vi "ACT_Loop.vi"() -> ()   [LabVIEW 2023, in "Intake_ACT.lvlib"]
uses:
  Intake_ACT.lvlib
  Cluster_CMD_ACT_Data.ctl
  ENUM_Shooter_Mode.ctl
  Cluster_Shooter Status.ctl
  Type Defs/Cluster_Speed Sensor Values.ctl
  Shooter/Cluster_Velocity Values.ctl
  Shooter/Cluster_Voltage Values.ctl
  ENUM_ACT_State.ctl
  <vilib>/Rock Robotics/WPI/MotorControl/WPI_MotorControlDeviceRef.ctl
  <vilib>/Rock Robotics/WPI/MotorControl/WPI_MotorControlType.ctl
  <vilib>/Rock Robotics/SystemInterfaces/DIO/FPGA_DIOPWMChannel.ctl
  <vilib>/Rock Robotics/WPI/PWM/WPI_PWMDeadband.ctl
  <vilib>/Rock Robotics/SystemInterfaces/DIO/FPGA_DIOChannel.ctl
  <vilib>/Rock Robotics/WPI/ThirdParty/Phoenix-LabVIEW/Motor Controller/Controls/CTRE_Phoenix_MotorControl_ControlMode.ctl
  ENUM_ACT_Action.ctl
  <vilib>/Rock Robotics/WPI/ThirdParty/Phoenix-LabVIEW/Motor Controller/Controls/CTRE_Phoenix_MotorControl_TalonFXInvertType.ctl
  <vilib>/Rock Robotics/WPI/ThirdParty/Phoenix-LabVIEW/Motor Controller/Controls/CTRE_Phoenix_MotorControl_NeutralMode.ctl
  RoboRIO Utilities/Global_STOP.vi
  Global_CMD_ACT_Data In.vi
  Global_ACT_Data Out.vi
  Shooter/Shooter_ACT.lvlib
panel:
  out "Motor Status":T1
  out "Target RPM":dbl
  out "Input DBL Data":T5
  out "Output DBL Data":dbl
  out "Cycle Time (S)":dbl format="%.3g"
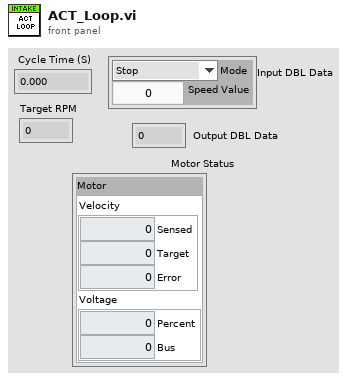
[diagram p1: front panel]
types:
  T1 = typedef "Intake_ACT.lvlib/Cluster_Shooter Status.ctl" = cluster{"Motor":T2}
  T2 = typedef "Cluster_Speed Sensor Values.ctl" = cluster{"Velocity":T3, "Voltage":T4}
  T3 = typedef "Shooter_ACT.lvlib/Cluster_Velocity Values.ctl" = cluster{"Sensed":dbl, "Target":dbl, "Error":dbl}
  T4 = typedef "Shooter_ACT.lvlib/Cluster_Voltage Values.ctl" = cluster{"Percent":dbl, "Bus":dbl}
  T5 = typedef "Intake_ACT.lvlib/Cluster_CMD_ACT_Data.ctl" = cluster{"Mode":T6, "Speed Value":dbl}
  T6 = typedef "Intake_ACT.lvlib/ENUM_Shooter_Mode.ctl" = enum16{"Stop", "Speed Percent", "Speed RPM"}
  T7 = typedef "CTRE_Phoenix_MotorControl_ControlMode.ctl" = u16
  T8 = typedef "WPI_MotorControlDeviceRef.ctl" = cluster{"DeviceStatus":errorcluster, "Type":T9, "PWM":cluster{"PWM Channel":T10, "DeadBand":T11}, "CAN":cluster{"Device Number":u8, "SetOutput VI Ref":variant, "GetOutput VI Ref":variant, "Enable VI Ref":variant, "Disable VI Ref":variant, "Data":variant}, "Invert":bool, "DIO PWM":cluster{"PWM \"Enable\" Channel":T10, "DIOChannel":T12, "PWM Rate":dbl}}
  T9 = typedef "WPI_MotorControlType.ctl" = enum16{"PWM", "CAN", "DIO PWM"}
  T10 = typedef "FPGA_DIOPWMChannel.ctl" = enum8{"PWM 0", "PWM 1", "PWM 2", "PWM 3", "PWM 4", "PWM 5", "PWM 6", "PWM 7", "PWM 8", "PWM 9", "PWM MXP 0", "PWM MXP 1", "PWM MXP 2", "PWM MXP 3", "PWM MXP 4", "PWM MXP 5", "PWM MXP 6", "PWM MXP 7", "PWM MXP 8", "PWM MXP 9", "Invalid"}
  T11 = typedef "WPI_PWMDeadband.ctl" = cluster{"Name":string, "maxPositivePwm":i32, "minPositivePwm":i32, "centerPwm":i32, "maxNegativePwm":i32, "minNegativePwm":i32, "angularRange":u16}
  T12 = typedef "FPGA_DIOChannel.ctl" = enum8{"DIO 0", "DIO 1", "DIO 2", "DIO 3", "DIO 4", "DIO 5", "DIO 6", "DIO 7", "DIO 8", "DIO 9", "DIO MXP 0", "DIO MXP 1", "DIO MXP 2", "DIO MXP 3", "DIO MXP 4", "DIO MXP 5", "DIO MXP 6", "DIO MXP 7", "DIO MXP 8", "DIO MXP 9", "DIO MXP 10", "DIO MXP 11", "DIO MXP 12", "DIO MXP 13", "DIO MXP 14", "DIO MXP 15", "SPI Port CS1", "SPI Port CS2", "SPI Port CS3", "SPI Port MISO", "SPI Port MOSI", "Invalid"}
  T13 = typedef "Intake_ACT.lvlib/ENUM_ACT_State.ctl" = enum16{"Starting", "Stopping", "Intaking", "Shutdown"}
  T14 = typedef "Intake_ACT.lvlib/ENUM_ACT_Action.ctl" = enum16{"No Action", "Reset Time", "Reset All", "Setup Motors", "Setup Sensors", "Stop", "Set Speed RPM", "Set Speed Percent"}
  T15 = cluster{"Motor Ref":T8, "State":T13, "Previous State":T13, "Current Time":timestamp, "Previous Time":timestamp, "Start Time":timestamp, "Target Time (ms)":u32, "Cycle Time(S)":dbl, "ACT Input":T5, "Motor Value":dbl, "Control Mode":T7, "Target RPM":dbl, "Motor Status":T1, "ACT Input from Shooter":T5}
  T16 = typedef "CTRE_Phoenix_MotorControl_NeutralMode.ctl" = enum8{"EEPROMSetting", "Override to Coast", "Override to Brake"}
  T17 = typedef "CTRE_Phoenix_MotorControl_TalonFXInvertType.ctl" = enum16{"Counter-Clockwise", "Clockwise"}
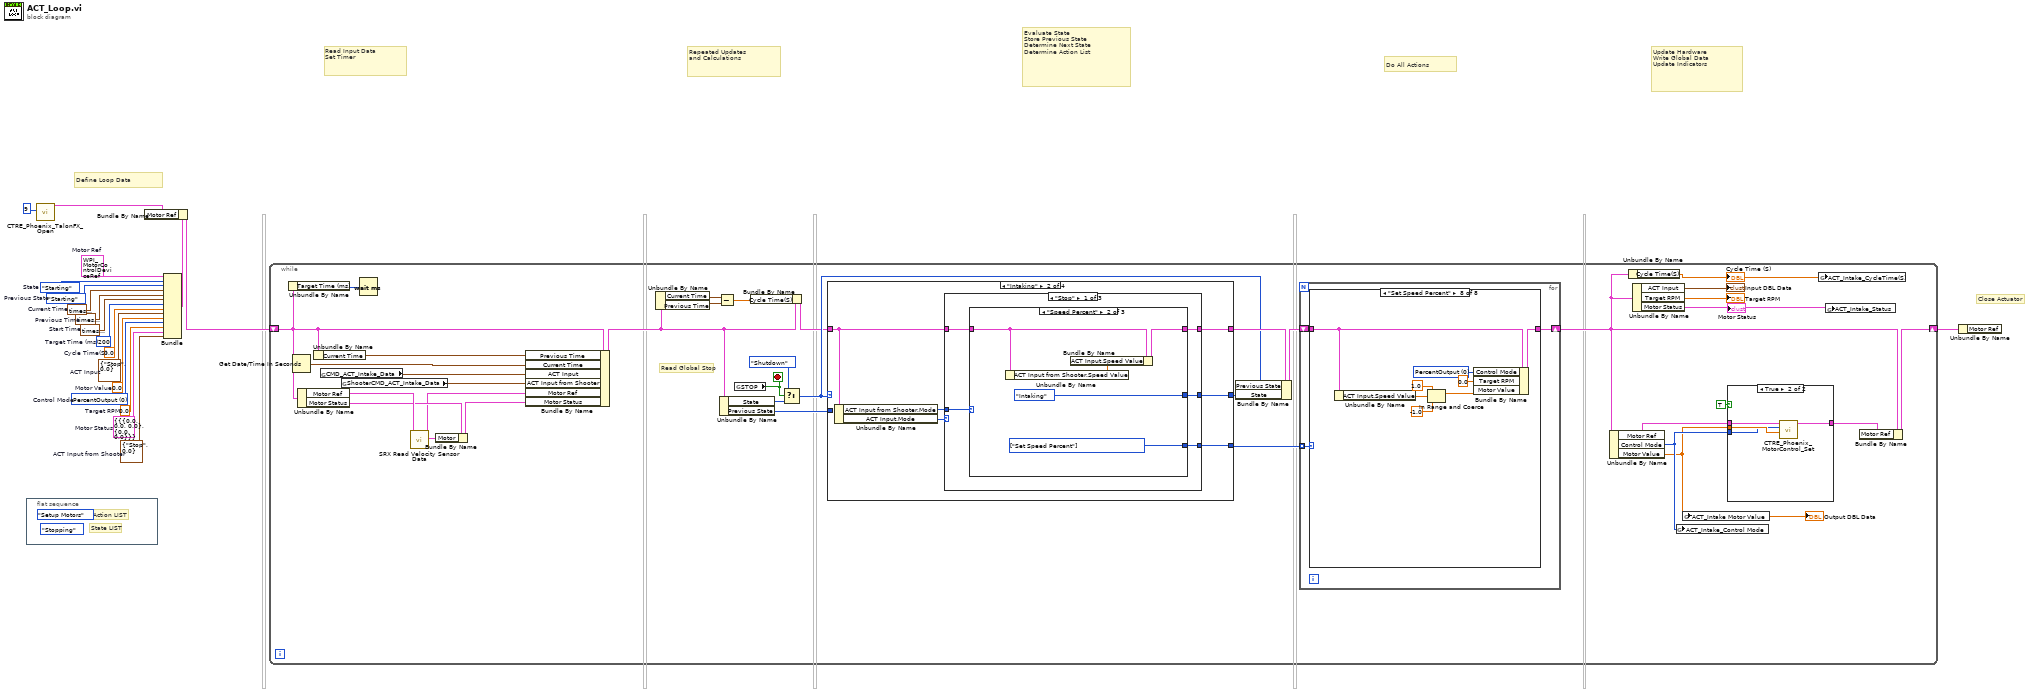
[diagram p0: block diagram]
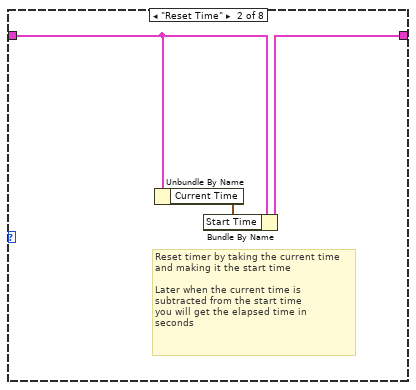
[diagram p4: hidden frame]
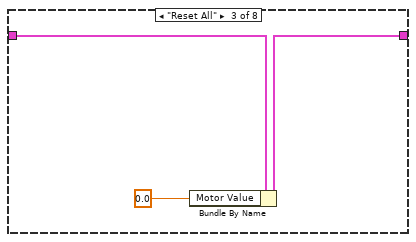
[diagram p5: hidden frame]
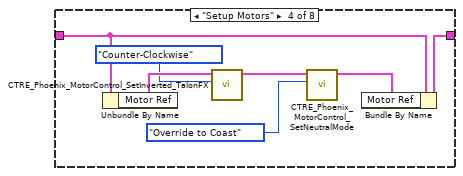
[diagram p6: hidden frame]
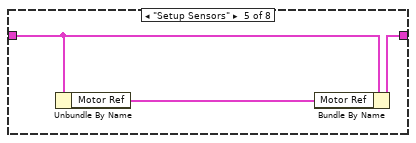
[diagram p7: hidden frame]
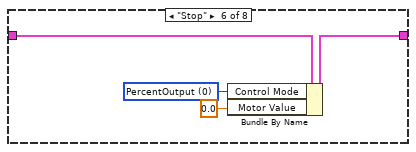
[diagram p8: hidden frame]
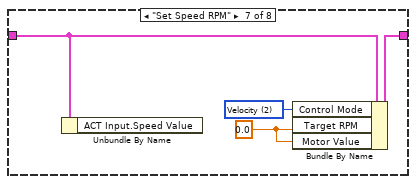
[diagram p9: hidden frame]
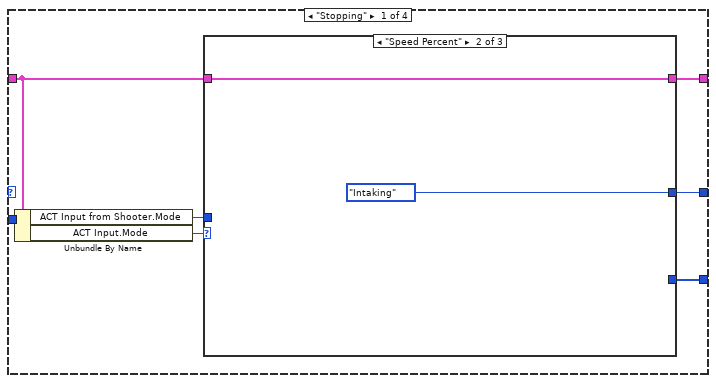
[diagram p10: hidden frame]
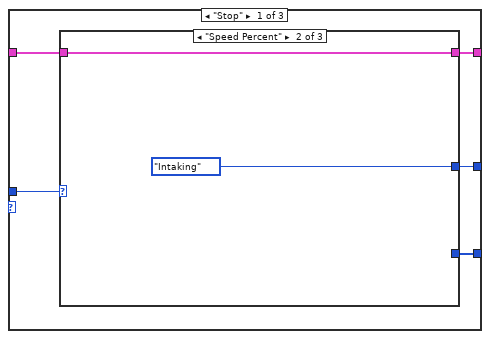
[diagram p11: hidden frame]
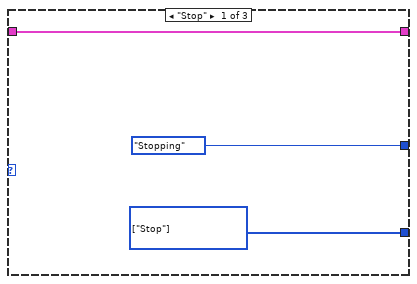
[diagram p12: hidden frame]
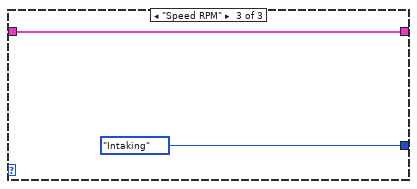
[diagram p13: hidden frame]
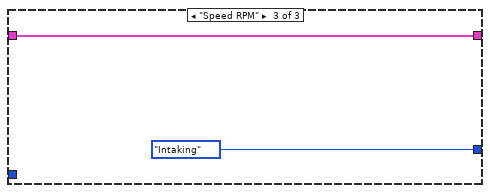
[diagram p14: hidden frame]
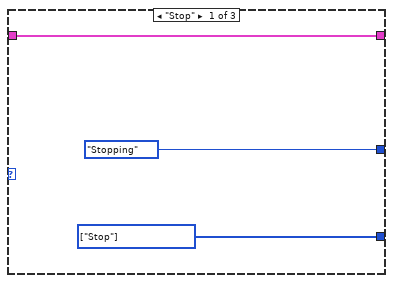
[diagram p15: hidden frame]
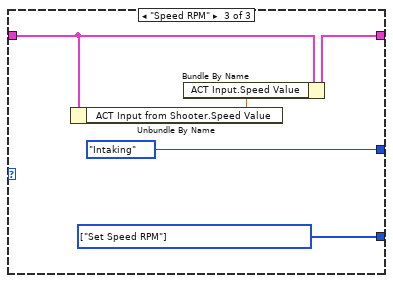
[diagram p16: hidden frame]
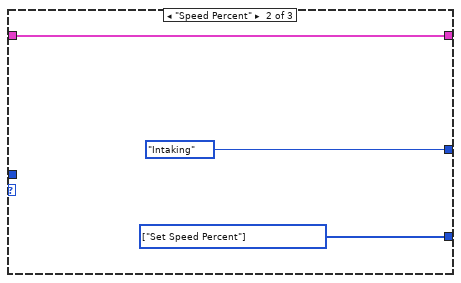
[diagram p17: hidden frame]
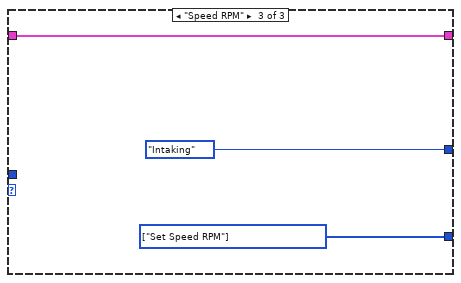
[diagram p18: hidden frame]
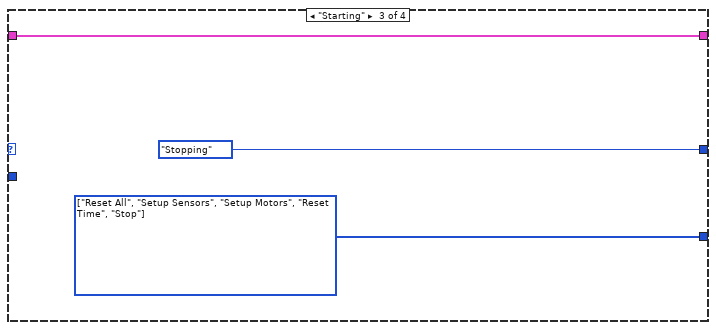
[diagram p19: hidden frame]
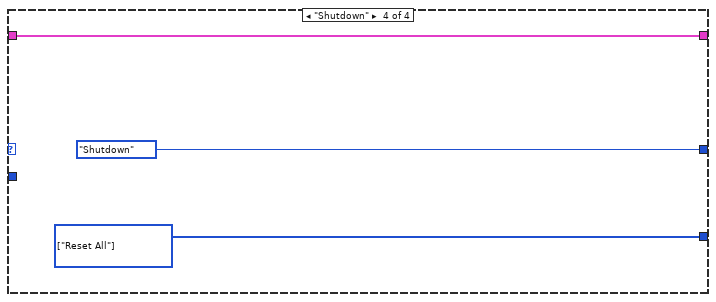
[diagram p20: hidden frame]
diagram:
  w1 = T5 {"Mode"=enum."Stop", "Speed Value"=0.0}  # ACT Input from Shooter
  w2 = T7 0 items=["PercentOutput"=0, "Position"=1, "Velocity"=2, "Current"=3, "Follower"=5, "MotionProfile"=6, "MotionMagic"=7, "MotionProfileArc"=10, "Disabled"=15]  # Control Mode
  w5 = T1 {"Motor"={"Velocity"={"Sensed"=0.0, "Target"=0.0, "Error"=0.0}, "Voltage"={"Percent"=0.0, "Bus"=0.0}}}  # Motor Status
  w6 = 0.0  # Target RPM
  w7 = T8 {"DeviceStatus"={"status"=FALSE, "code"=0, "source"=""}, "Type"=enum."PWM", "PWM"={"PWM Channel"=enum."PWM 1", "DeadBand"={"Name"="", "maxPositivePwm"=0, "minPositivePwm"=0, "centerPwm"=0, "maxNegativePwm"=0, "minNegativePwm"=0, "angularRange"=0}}, "CAN"={"Device Number"=0, "SetOutput VI Ref"=variant(enum8{"Percent VBus", "Current", "Speed", "Position", "Voltage"} enum."Percent VBus"), "GetOutput VI Ref"=variant(refnum<k1> refnum), "Enable VI Ref"=variant(dbl 12.0), "Disable VI Ref"=variant(enum8{"Percent VBus", "Speed", "Position", "Slave", "Unchanged / Invalid", "Voltage Compensation", "Current", "Motion Profile"} enum."Percent VBus"), "Data"=variant}, "Invert"=FALSE, "DIO PWM"={"PWM \"Enable\" Channel"=enum."Invalid", "DIOChannel"=enum."Invalid", "PWM Rate"=0.0}}  # Motor Ref
  w11 = 0.0  # Cycle Time(S)
  w12 = ENUM_ACT_State."Starting"  # Previous State
  w13 = timestamp(0 s since 1904-01-01)  # Previous Time
  w14 = u32 200  # Target Time (ms)
  w15 = 0.0  # Motor Value
  w16 = T5 {"Mode"=enum."Stop", "Speed Value"=0.0}  # ACT Input
  w17 = timestamp(0 s since 1904-01-01)  # Start Time
  w18 = timestamp(0 s since 1904-01-01)  # Current Time
  w19 = ENUM_ACT_State."Starting"  # State
  # "Close Actuator"
  # "Define Loop Data"
  # "Repeated Updates\nand Calculations"
  # "Read Input Data\nSet Timer"
  # "Evaluate State\nStore Previous State\nDetermine Next State\nDetermine Action List"
  # "Do All Actions"
  # "Update Hardware\nWrite Global Data\nUpdate Indicators"
  n1 = flat-sequence {
    frame #0 {
      (unwired) ENUM_ACT_State."Stopping" ("State")
      (unwired) ENUM_ACT_Action."Setup Motors" ("Action")
      # "State LIST"
      # "Action LIST"
    }
  }
  n2 = call <vilib>:"CTRE_Phoenix_TalonFX_Open.vi"("Device Number"=u8 9) -> ("PhoenixMotorControlDevRef"=w4:T8)  [unwired: 9 in, 1 out]
  n3 = Bundle("Motor Ref"=w7, "State"=w19, "Previous State"=w12, "Current Time"=w18, "Previous Time"=w13, "Start Time"=w17, "Target Time (ms)"=w14, "Cycle Time(S)"=w11, "ACT Input"=w16, "Motor Value"=w15, "Control Mode"=w2, "Target RPM"=w6, "Motor Status"=w5, "ACT Input from Shooter"=w1) -> (w9:T15)  [unwired: 1 in]
  n4 = Bundle By Name(cluster=w9, "Motor Ref"=w4) -> (w8:T15)
  n5 = while {
    shift-right: [w35] -> w10
    shift-left: w8 -> [w28]
    stop <- w51 stop-if-true
    # "Read Global Stop"
    n6 = Unbundle By Name(w28) -> ("Target Time (ms)"=w48:u32)
    n7 = Get Date/Time In Seconds() -> (seconds since 1Jan1904=w55:timestamp)
    n8 = Unbundle By Name(w28) -> ("Motor Ref"=w27:T8, "Motor Status"=w26:T1)
    n9 = Unbundle By Name(w28) -> ("Current Time"=w47:timestamp)
    n10 = global read "Global_CMD_ACT_Data In.vi" "CMD_ACT_Intake_Data"() -> (w37:T5)
    n11 = global read "Global_CMD_ACT_Data In.vi" "ShooterCMD_ACT_Intake_Data"() -> (w20:T5)
    n12 = Wait (ms)(milliseconds to wait=w48) -> ()  [unwired: 1 out]
    n13 = call "SRX Read Velocity Sensor Data.vi"("SRX Ref"=w27) -> ("Sensor Status Out"=w21:T2, "SRX Ref Out"=w24:T8)  [unwired: 8 in, 1 out]
    n14 = Bundle By Name(cluster=w26, "Motor"=w21) -> (w25:T1)
    n15 = Bundle By Name(cluster=w28, "Previous Time"=w47, "Current Time"=w55, "ACT Input"=w37, "ACT Input from Shooter"=w20, "Motor Ref"=w24, "Motor Status"=w25) -> (w42:T15)
    n16 = Unbundle By Name(w42) -> ("Current Time"=w43:timestamp, "Previous Time"=w44:timestamp)
    n17 = Subtract(x=w43, y=w44) -> (x-y=w40:dbl)
    n18 = Unbundle By Name(w42) -> ("State"=w49:T13, "Previous State"=w46:T13)
    n19 = global read "Global_STOP.vi" "STOP"() -> (w51:bool)
    n20 = Bundle By Name(cluster=w42, "Cycle Time(S)"=w40) -> (w41:T15)
    n21 = Select(t=ENUM_ACT_State."Shutdown" ("State"), s=w51, f=w49) -> (s? t:f=w45:T13)
    n22 = case shown="\"Intaking\"" w45 {
      tunnel: w41 -> [w98 w121 w151 w154]
      tunnel: [w97 w120 w151 w154] -> w53
      tunnel: [w101 w123 ENUM_ACT_State."Stopping" ("State") ENUM_ACT_State."Shutdown" ("State")] -> w52
      tunnel: [w102 w124 w149 w152] -> w39
      tunnel: w46 -> [_ _ _ _]
      frame "Stopping" {
        n23 = Unbundle By Name(w98) -> ("ACT Input from Shooter.Mode"=w99:T6, "ACT Input.Mode"=w100:T6)
        n24 = case shown="\"Speed Percent\"" w100 {
          tunnel: [w107 _ _] -> w102
          tunnel: [w106 ENUM_ACT_State."Intaking" ("State") ENUM_ACT_State."Intaking" ("State")] -> w101
          tunnel: w99 -> [w103 _ _]
          tunnel: w98 -> [w105 w115 w117]
          tunnel: [w104 w115 w117] -> w97
          frame "Stop" {
            n25 = case shown="\"Speed Percent\"" w103 {
              tunnel: [w108 _ _] -> w107
              tunnel: [ENUM_ACT_State."Stopping" ("State") ENUM_ACT_State."Intaking" ("State") ENUM_ACT_State."Intaking" ("State")] -> w106
              tunnel: w105 -> [w110 w111 w113]
              tunnel: [w110 w111 w113] -> w104
              frame "Stop" {
                w108 = T14[] [enum."Stop"] items=["No Action", "Reset Time", "Reset All", "Setup Motors", "Setup Sensors", "Stop", "Set Speed RPM", "Set Speed Percent"] ("Actions")
              }
              frame "Speed Percent" {
              }
              frame "Speed RPM" {
              }
            }
          }
          frame "Speed Percent" {
          }
          frame "Speed RPM" {
          }
        }
      }
      frame "Intaking" {
        n26 = Unbundle By Name(w121) -> ("ACT Input from Shooter.Mode"=w119:T6, "ACT Input.Mode"=w122:T6)
        n27 = case shown="\"Stop\"" w122 {
          tunnel: [w128 w144 w147] -> w124
          tunnel: [w129 ENUM_ACT_State."Intaking" ("State") ENUM_ACT_State."Intaking" ("State")] -> w123
          tunnel: w121 -> [w126 w143 w146]
          tunnel: [w125 w143 w146] -> w120
          tunnel: w119 -> [w127 _ _]
          frame "Stop" {
            n28 = case shown="\"Speed Percent\"" w127 {
              tunnel: [ENUM_ACT_State."Stopping" ("State") ENUM_ACT_State."Intaking" ("State") ENUM_ACT_State."Intaking" ("State")] -> w129
              tunnel: [w131 w136 w141] -> w128
              tunnel: w126 -> [w130 w134 w139]
              tunnel: [w130 w135 w140] -> w125
              frame "Stop" {
                w131 = T14[] [enum."Stop"] items=["No Action", "Reset Time", "Reset All", "Setup Motors", "Setup Sensors", "Stop", "Set Speed RPM", "Set Speed Percent"] ("Actions")
              }
              frame "Speed Percent" {
                w136 = T14[] [enum."Set Speed Percent"] items=["No Action", "Reset Time", "Reset All", "Setup Motors", "Setup Sensors", "Stop", "Set Speed RPM", "Set Speed Percent"] ("Actions")
                n29 = Unbundle By Name(w134) -> ("ACT Input from Shooter.Speed Value"=w133:dbl)
                n30 = Bundle By Name(cluster=w134, "ACT Input.Speed Value"=w133) -> (w135:T15)
              }
              frame "Speed RPM" {
                w141 = T14[] [enum."Set Speed RPM"] items=["No Action", "Reset Time", "Reset All", "Setup Motors", "Setup Sensors", "Stop", "Set Speed RPM", "Set Speed Percent"] ("Actions")
                n31 = Unbundle By Name(w139) -> ("ACT Input from Shooter.Speed Value"=w138:dbl)
                n32 = Bundle By Name(cluster=w139, "ACT Input.Speed Value"=w138) -> (w140:T15)
              }
            }
          }
          frame "Speed Percent" {
            w144 = T14[] [enum."Set Speed Percent"] items=["No Action", "Reset Time", "Reset All", "Setup Motors", "Setup Sensors", "Stop", "Set Speed RPM", "Set Speed Percent"] ("Actions")
          }
          frame "Speed RPM" {
            w147 = T14[] [enum."Set Speed RPM"] items=["No Action", "Reset Time", "Reset All", "Setup Motors", "Setup Sensors", "Stop", "Set Speed RPM", "Set Speed Percent"] ("Actions")
          }
        }
      }
      frame "Starting" {
        w149 = T14[] [enum."Reset All", enum."Setup Sensors", enum."Setup Motors", enum."Reset Time", enum."Stop"] items=["No Action", "Reset Time", "Reset All", "Setup Motors", "Setup Sensors", "Stop", "Set Speed RPM", "Set Speed Percent"] ("Actions")
      }
      frame "Shutdown" {
        w152 = T14[] [enum."Reset All"] items=["No Action", "Reset Time", "Reset All", "Setup Motors", "Setup Sensors", "Stop", "Set Speed RPM", "Set Speed Percent"] ("Actions")
      }
    }
    n33 = Bundle By Name(cluster=w53, "Previous State"=w45, "State"=w52) -> (w54:T15)
    n34 = for {
      tunnel: w39 -> [w63] mode=indexing
      shift-right: [w62] -> w36
      shift-left: w54 -> [w61]
      n35 = case shown="\"Set Speed Percent\"" w63 {
        tunnel: w61 -> [w64 w67 w70 w77 w80 w83 w87 w95]
        tunnel: [w64 w66 w69 w76 w79 w84 w88 w96] -> w62
        frame "No Action" {
        }
        frame "Reset Time" {
          # "Reset timer by taking the current time\nand making it the start time\n\nLater when the current time is \nsubtracted from the start time\nyou will get the elapsed time in \nseconds"
          n36 = Unbundle By Name(w67) -> ("Current Time"=w65:timestamp)
          n37 = Bundle By Name(cluster=w67, "Start Time"=w65) -> (w66:T15)
        }
        frame "Reset All" {
          n38 = Bundle By Name(cluster=w70, "Motor Value"=0.0 ("FG Write Value")) -> (w69:T15)
        }
        frame "Setup Motors" {
          n39 = Unbundle By Name(w77) -> ("Motor Ref"=w73:T8)
          n40 = call <vilib>:"CTRE_Phoenix_MotorControl_SetInverted_TalonFX.vi"("Invert Type"=CTRE_Phoenix_MotorControl_TalonFXInvertType."Counter-Clockwise", "PhoenixMotorControlDevRef"=w73) -> ("PhoenixMotorControlDevRef"=w74:T8)  [unwired: 8 in, 1 out]
          n41 = call <vilib>:"CTRE_Phoenix_MotorControl_SetNeutralMode.vi"("Motor Control Neutral Mode"=CTRE_Phoenix_MotorControl_NeutralMode."Override to Coast", "PhoenixMotorControlDevRef"=w74) -> ("PhoenixMotorControlDevRef"=w75:T8)  [unwired: 8 in, 1 out]
          n42 = Bundle By Name(cluster=w77, "Motor Ref"=w75) -> (w76:T15)
        }
        frame "Setup Sensors" {
          n43 = Unbundle By Name(w80) -> ("Motor Ref"=w78:T8)
          n44 = Bundle By Name(cluster=w80, "Motor Ref"=w78) -> (w79:T15)
        }
        frame "Stop" {
          w81 = T7 0 items=["PercentOutput"=0, "Position"=1, "Velocity"=2, "Current"=3, "Follower"=5, "MotionProfile"=6, "MotionMagic"=7, "MotionProfileArc"=10, "Disabled"=15] ("Control Mode")
          n45 = Bundle By Name(cluster=w83, "Control Mode"=w81, "Motor Value"=0.0) -> (w84:T15)
        }
        frame "Set Speed RPM" {
          w85 = 0.0 ("Target RPM")
          w86 = T7 2 items=["PercentOutput"=0, "Position"=1, "Velocity"=2, "Current"=3, "Follower"=5, "MotionProfile"=6, "MotionMagic"=7, "MotionProfileArc"=10, "Disabled"=15] ("Control Mode")
          n46 = Unbundle By Name(w87) -> ()  [unwired: 1 out]
          n47 = Bundle By Name(cluster=w87, "Control Mode"=w86, "Target RPM"=w85, "Motor Value"=w85) -> (w88:T15)
        }
        frame "Set Speed Percent" {
          w89 = T7 0 items=["PercentOutput"=0, "Position"=1, "Velocity"=2, "Current"=3, "Follower"=5, "MotionProfile"=6, "MotionMagic"=7, "MotionProfileArc"=10, "Disabled"=15] ("Control Mode")
          n48 = Unbundle By Name(w95) -> ("ACT Input.Speed Value"=w93:dbl)
          n49 = In Range and Coerce(upper limit=1.0, x=w93, lower limit=-1.0 ("upper limit")) -> (coerced(x)=w90:dbl)  [unwired: 1 out]
          n50 = Bundle By Name(cluster=w95, "Control Mode"=w89, "Target RPM"=0.0, "Motor Value"=w90) -> (w96:T15)
        }
      }
    }
    n51 = Unbundle By Name(w36) -> ("Motor Ref"=w33:T8, "Control Mode"=w31:T7, "Motor Value"=w30:dbl)
    "Output DBL Data" <- w30
    n52 = Unbundle By Name(w36) -> ("Cycle Time(S)"=w34:dbl)
    "Cycle Time (S)" <- w34
    n53 = Unbundle By Name(w36) -> ("ACT Input"=→"Input DBL Data":T5, "Target RPM"=→"Target RPM":dbl, "Motor Status"=w23:T1)
    "Motor Status" <- w23
    n54 = global write "Global_ACT_Data Out.vi" "ACT_Intake_Control Mode"(w31) -> ()
    n55 = global write "Global_ACT_Data Out.vi" "ACT_Intake Motor Value"(w30) -> ()
    n56 = case shown="True" TRUE {
      tunnel: w33 -> [w56 w60]
      tunnel: [w56 w59] -> w32
      tunnel: w31 -> [_ w57]
      tunnel: w30 -> [_ w58]
      frame False {
      }
      frame True {
        n57 = call <vilib>:"CTRE_Phoenix_MotorControl_Set.vi"("Output"=w58, "Control Mode"=w57, "PhoenixMotorControlDevRef"=w60) -> ("PhoenixMotorControlDevRef"=w59:T8)  [unwired: 7 in, 1 out]
      }
    }
    n58 = global write "Global_ACT_Data Out.vi" "ACT_Intake_CycleTime(S)"(w34) -> ()
    n59 = global write "Global_ACT_Data Out.vi" "ACT_Intake_Status"(w23) -> ()
    n60 = Bundle By Name(cluster=w36, "Motor Ref"=w32) -> (w35:T15)
  }
  n61 = Unbundle By Name(w10) -> ()  [unwired: 1 out]
